vi "GUI.SetValue.vi"(6 "timeout (ms)":i32, 8 "error in (no error)":errorcluster, 10 "Value":T1, 11 "GUI":refnum<class "GUI.lvclass">) -> (0 "error out":errorcluster, 3 "GUI out":refnum<class "GUI.lvclass">, 4 "timed out?":bool)   [LabVIEW 2022 SP3, in "GUI.lvclass"]
doc: "---------------------------------------------------------------\nJKI State Machine Objects™\nhttp://jki.net/state-machine-objects/\nCopyright (C) 2005-2015, JKI <info@jki.net>\nALL RIGHTS RESERVEDJKI State Machine Objects (SMO) 1.0.0.5\nJKI - JKI\nCopyright (c) 2016, JKI"
uses:
  GUI.lvclass
  C:/Program Files (x86)/National Instruments/LabVIEW 2022/vi.lib/JKI/JKI SMO/SMO/SMO.lvclass
  Typedefs/Value.ctl
  Typedefs/NewValueEvent--Cluster.ctl
  <vilib>/JKI/JKI SMO/SMO/SMO.lvclass/SMO.ctl
  <vilib>/JKI/JKI SMO/SMO/Private/ReftoDVR--SMO.vi
  <vilib>/JKI/JKI SMO/SMO/SMO.lvclass
panel:
  # "For instructions on how to use the JKI State Machine Objects, examples and video tutorials, visit:\nhttp://jki.net/state-machine-objects/\n\nJKI State Machine Objects™\nhttp://jki.net/state-machine-objects/\nCopyright (C) 2005-2015, JKI <info@jki.net>\nALL RIGHTS RESERVED"
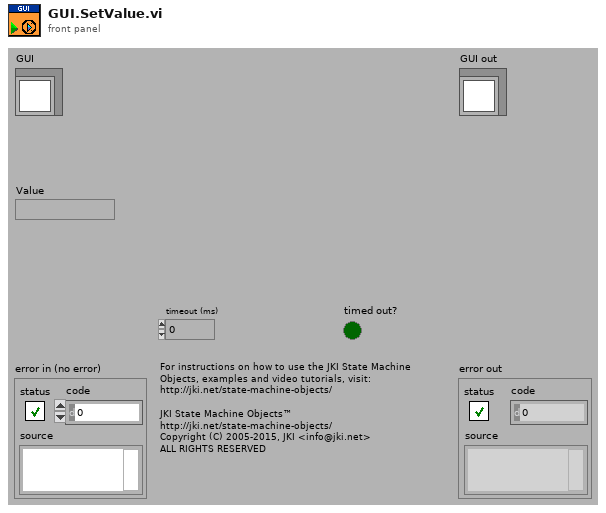
[diagram p1: front panel]
types:
  T1 = typedef "GUI.lvclass/Value.ctl" = string
  T2 = typedef "SMO.lvclass/SMOState --Enum.ctl" = enum16{"unknown", "Created", "Started", "Stopped"}
  T3 = typedef "GUI.lvclass/NewValueEvent--Cluster.ctl" = cluster{"Value":string}
  T4 = typedef "SMO.lvclass/Public Events.ctl" = cluster{"Error":refnum<user-event>, "State":refnum<user-event>, "Reserve State":refnum<user-event>}
  T5 = typedef "GUI.lvclass/PublicEvents--Cluster.ctl" = cluster{"Value Changed":refnum<user-event>}
  T6 = typedef "GUI.lvclass/PrivateEvents--Cluster.ctl" = cluster{"New Value":refnum<user-event>}
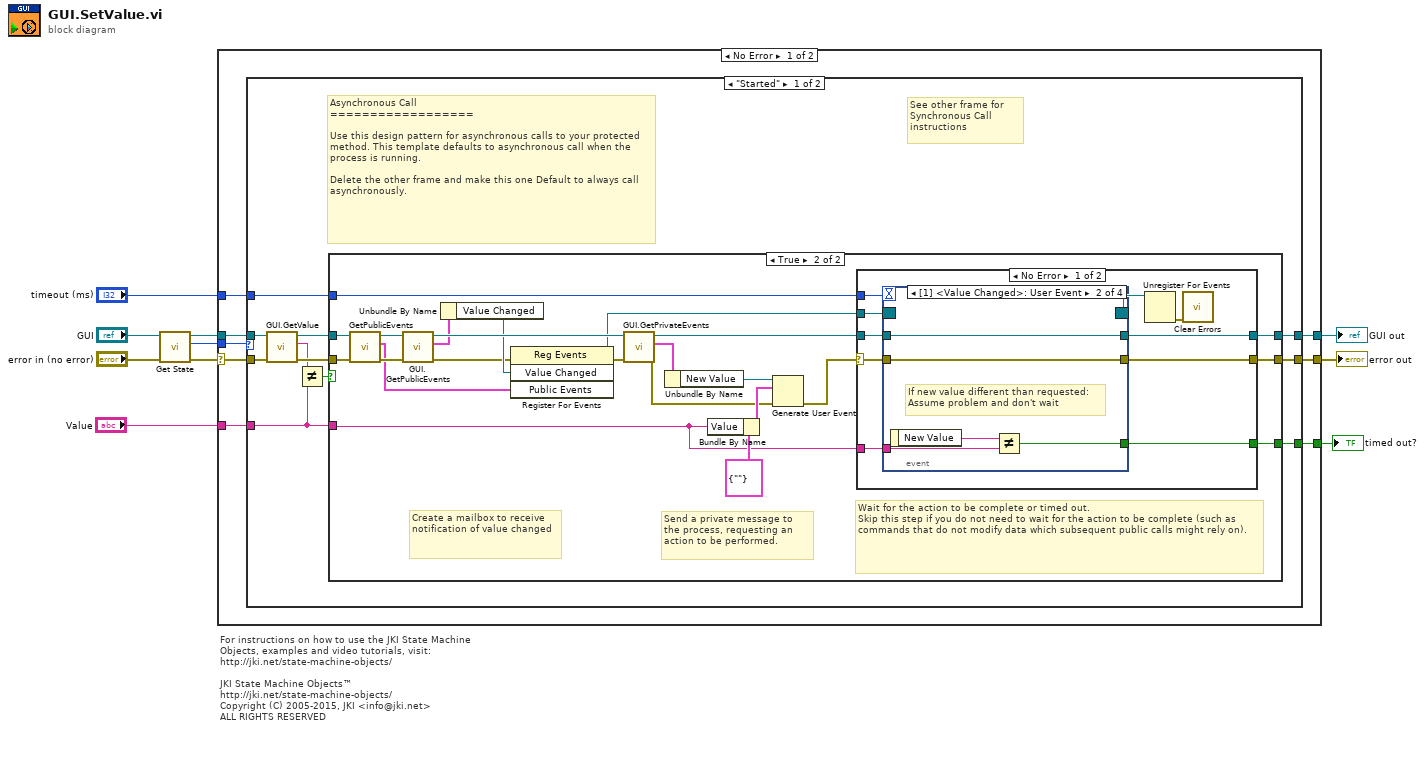
[diagram p0: block diagram]
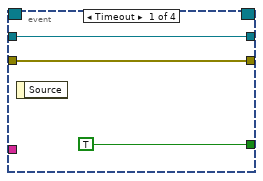
[diagram p3: hidden frame]
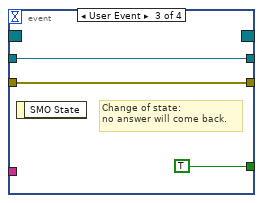
[diagram p4: hidden frame]
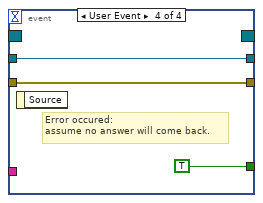
[diagram p5: hidden frame]
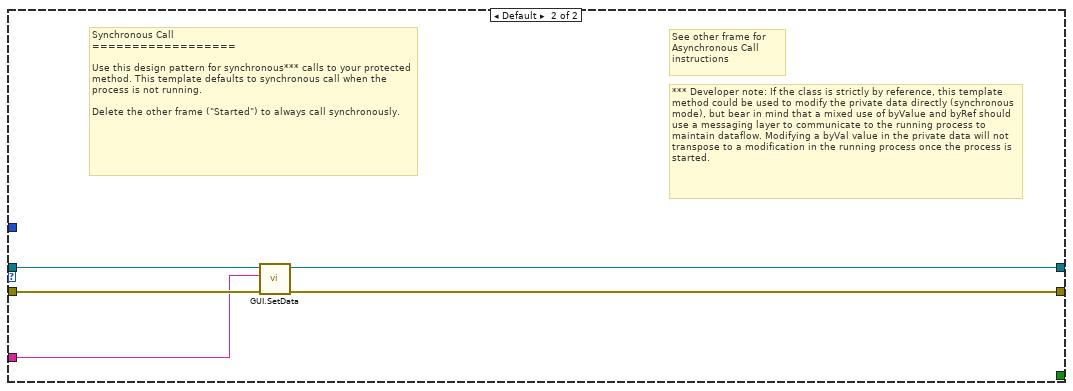
[diagram p7: hidden frame]
diagram:
  # "For instructions on how to use the JKI State Machine Objects, examples and video tutorials, visit:\nhttp://jki.net/state-machine-objects/\n\nJKI State Machine Objects™\nhttp://jki.net/state-machine-objects/\nCopyright (C) 2005-2015, JKI <info@jki.net>\nALL RIGHTS RESERVED"
  n1 = call <vilib>:"Get State.vi"("error in (no error)"="error in (no error)", "SMO"="GUI") -> ("error out"=w4:errorcluster, "SMO State"=w3:T2, "SMO out"=w6:refnum<class "GUI.lvclass">)  [unwired: 7 in]
  n2 = case shown="No Error" w4 {
    selector: w4 -> [w17 w86]
    tunnel: w6 -> [w14 w87]
    tunnel: [w16 w86] -> w10
    tunnel: [w15 w87] -> w9
    tunnel: "Value" -> [w18 _]
    tunnel: w3 -> [w13 _]
    tunnel: "timeout (ms)" -> [w12 _]
    tunnel: [w11 _] -> w1
    frame No Error {
      n3 = case shown="\"Started\"" w13 {
        tunnel: w18 -> [w23 w82]
        tunnel: w17 -> [w27 w83]
        tunnel: [w20 w81] -> w16
        tunnel: [w21 w84] -> w15
        tunnel: w14 -> [w29 w85]
        tunnel: w12 -> [w22 _]
        tunnel: [w19 _] -> w11
        frame "Started" {
          # "See other frame for\nSynchronous Call\ninstructions"
          # "Asynchronous Call\n==================\n\nUse this design pattern for asynchronous calls to your protected method. This template defaults to asynchronous call when the process is running.\n\nDelete the other frame and make this one Default to always call asynchronously."
          n4 = call "GUI.GetValue.vi"("error in (no error)"=w27, "GUI"=w29) -> ("error out"=w26:errorcluster, "Value"=w24:T1, "GUI out"=w28:refnum<class "GUI.lvclass">)  [unwired: 7 in]
          n5 = Not Equal?(x=w24, y=w23) -> (x != y?=w25:bool)
          n6 = case shown="True" w25 {
            tunnel: w28 -> [w31 w38]
            tunnel: w26 -> [w30 w36]
            tunnel: w23 -> [_ w32]
            tunnel: w22 -> [_ w45]
            tunnel: [w31 w40] -> w21
            tunnel: [w30 w41] -> w20
            tunnel: [_ w39] -> w19
            frame False {
              # "Already same value: No Op"
            }
            frame True {
              # "Wait for the action to be complete or timed out.\nSkip this step if you do not need to wait for the action to be complete (such as commands that do not modify data which subsequent public calls might rely on)."
              # "Send a private message to the process, requesting an action to be performed."
              # "Create a mailbox to receive notification of value changed"
              n7 = call <vilib>:"GetPublicEvents.vi"("error in (no error)"=w36, "SMO"=w38) -> ("error out"=w35:errorcluster, "Public Events"=w34:T4, "SMO out"=w37:refnum<class "GUI.lvclass">)  [unwired: 7 in]
              n8 = call "GUI.GetPublicEvents.vi"("error in (no error)"=w35, "GUI"=w37) -> ("error out"=w47:errorcluster, "SMO.BasicByRef Public Events"=w49:T5, "GUI out"=w52:refnum<class "GUI.lvclass">)  [unwired: 7 in]
              n9 = Unbundle By Name(w49) -> ("Value Changed"=w48:refnum<user-event>)
              n10 = register-events(error in=w47, w48, w34) -> (reference out=w33:refnum<event-registration>, error out=w46:errorcluster)  [unwired: 1 in]
              n11 = call "GUI.GetPrivateEvents.vi"("error in (no error)"=w46, "GUI"=w52) -> ("error out"=w43:errorcluster, "Private Events"=w54:T6, "GUI out"=w44:refnum<class "GUI.lvclass">)  [unwired: 7 in]
              n12 = Unbundle By Name(w54) -> ("New Value"=w53:refnum<user-event>)
              n13 = Bundle By Name(cluster=T3 {"Value"=""} ("event data"), "Value"=w32) -> (w50:T3)
              n14 = Generate User Event(user event=w53, event data cluster=w50, error in=w43) -> (error out=w42:errorcluster)  [unwired: 1 in, 1 out]
              n15 = case shown="No Error" w42 {
                selector: w42 -> [w61 w80]
                tunnel: w45 -> [w64 _]
                tunnel: w44 -> [w63 w79]
                tunnel: [w60 w80] -> w41
                tunnel: [w62 w79] -> w40
                tunnel: [w59 _] -> w39
                tunnel: w33 -> [w58 _]
                tunnel: w32 -> [w55 _]
                frame No Error {
                  n16 = event shown="[1] <Value Changed>: User Event" {
                    selector: w58 -> [_ _ _ _]
                    dyn-events: [_ _ _ _] -> w57
                    timeout: w64 -> [_ _ _ _]
                    tunnel: w63 -> [w67 w72 w75 w78]
                    tunnel: [w67 w72 w75 w78] -> w62
                    tunnel: [w66 w71 w74 w77] -> w60
                    tunnel: w61 -> [w66 w71 w74 w77]
                    tunnel: [TRUE w69 TRUE TRUE] -> w59
                    tunnel: w55 -> [_ w68 _ _]
                    event Timeout {
                      n17 = event-data() -> ()  [unwired: 1 in, 1 out]
                    }
                    event User Event {
                      # "If new value different than requested:\nAssume problem and don't wait"
                      n18 = event-data() -> ("New Value"=w70:string)  [unwired: 1 in]
                      n19 = Not Equal?(x=w70, y=w68) -> (x != y?=w69:bool)
                    }
                    event User Event {
                      # "Change of state: \nno answer will come back."
                      n20 = event-data() -> ()  [unwired: 1 in, 1 out]
                    }
                    event User Event {
                      # "Error occured: \nassume no answer will come back."
                      n21 = event-data() -> ()  [unwired: 1 in, 1 out]
                    }
                  }
                  n22 = Unregister For Events(event registration refnum=w57) -> (error out=w56:errorcluster)  [unwired: 1 in]
                  n23 = call <vilib>:"Clear Errors.vi"("error in (no error)"=w56) -> ()  [unwired: 5 in, 2 out]
                }
                frame Error {
                }
              }
            }
          }
        }
        frame Default {
          # "*** Developer note: If the class is strictly by reference, this template method could be used to modify the private data directly (synchronous mode), but bear in mind that a mixed use of byValue and byRef should use a messaging layer to communicate to the running process to maintain dataflow. Modifying a byVal value in the private data will not transpose to a modification in the running process once the process is started."
          # "See other frame for\nAsynchronous Call\ninstructions"
          # "Synchronous Call\n==================\n\nUse this design pattern for synchronous*** calls to your protected method. This template defaults to synchronous call when the process is not running.\n\nDelete the other frame (\"Started\") to always call synchronously."
          n24 = call "GUI.SetData.vi"("error in (no error)"=w83, "Value"=w82, "GUI"=w85) -> ("error out"=w81:errorcluster, "GUI out"=w84:refnum<class "GUI.lvclass">)  [unwired: 7 in]
        }
      }
    }
    frame Error {
      # "Upstream error or State Machine Object has not been created."
    }
  }
  "error out" <- w10
  "GUI out" <- w9
  "timed out?" <- w1
